vi "create.from_set.vi"(8 "error in":errorcluster, 10 "labels":set{string}(c389)) -> (0 "error out":errorcluster, 3 "properties out":refnum<class "labels.lvclass">)   [LabVIEW 2020, in "nominal types.lvlib" / "labels.lvclass"]
uses:
  labels.lvclass
  labels.lvclass/labels.ctl
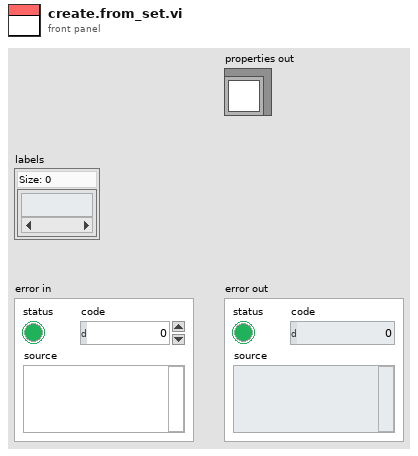
[diagram p1: front panel]
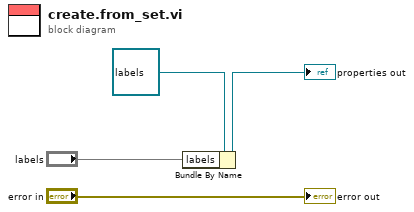
[diagram p0: block diagram]
diagram:
  n1 = Bundle By Name(cluster=refnum<class "labels.lvclass"> refnum ("properties out"), "labels"="labels") -> (→"properties out":refnum<class "labels.lvclass">)
  "error out" <- "error in"
